vi "Send Query.vi"(8 "error in (no error)":errorcluster, 9 "Bytes Count":u32=1024, 10 "write buffer":string, 11 "VISA resource name":refnum<visa-resource-name>) -> (0 "error out":errorcluster, 2 "read buffer":string, 3 "VISA resource name out":refnum<visa-resource-name>)   [LabVIEW 2023, in "Anritsu Power Meter.lvlib"]
uses:
  Anritsu Power Meter.lvlib
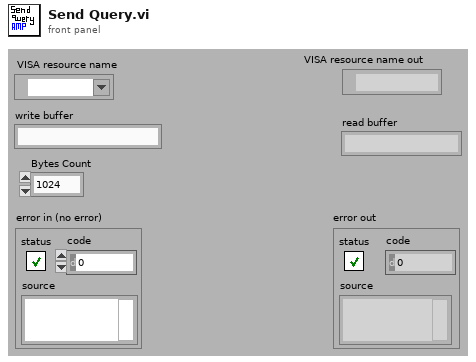
[diagram p1: front panel]
types:
  T1 = typedef "Semaphore RefNum" = refnum<k1>
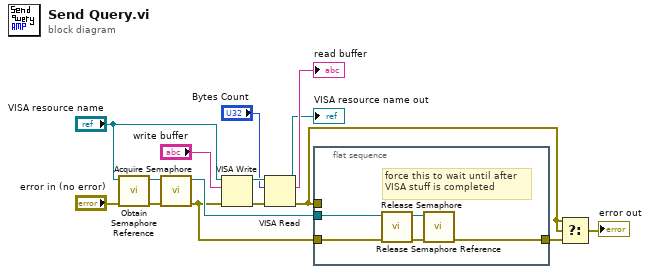
[diagram p0: block diagram]
diagram:
  n1 = call <vilib>:"Obtain Semaphore Reference.vi"("error in (no error)"="error in (no error)", "name (unnamed)"="VISA resource name") -> ("error out"=w10:errorcluster, "semaphore"=w11:T1)  [unwired: 1 in, 3 out]
  n2 = call <vilib>:"Acquire Semaphore.vi"("error in (no error)"=w10, "semaphore"=w11) -> ("error out"=w4:errorcluster, "semaphore out"=w8:T1)  [unwired: 1 in, 3 out]
  n3 = VISA Write(VISA resource name="VISA resource name", write buffer="write buffer", error in (no error)=w4) -> (VISA resource name out=w15:refnum<visa-resource-name>, error out=w13:errorcluster)  [unwired: 1 out]
  n4 = VISA Read(VISA resource name=w15, byte count="Bytes Count", error in (no error)=w13) -> (VISA resource name out=→"VISA resource name out":refnum<visa-resource-name>, read buffer=→"read buffer":string, error out=w3:errorcluster)  [unwired: 1 out]
  n5 = flat-sequence {
    tunnel: w8 -> [w20]
    tunnel: [w17] -> w5
    tunnel: w4 -> [w16]
    tunnel: w3 -> [_]
    frame #0 {
      # "force this to wait until after \nVISA stuff is completed"
      n6 = call <vilib>:"Release Semaphore.vi"("error in (no error)"=w16, "semaphore"=w20) -> ("error out"=w18:errorcluster, "semaphore out"=w19:T1)  [unwired: 4 out]
      n7 = call <vilib>:"Release Semaphore Reference.vi"("error in (no error)"=w18, "semaphore"=w19) -> ("error out"=w17:errorcluster)  [unwired: 9 out]
    }
  }
  n8 = Select(t=w3, s=w3, f=w5) -> (s? t:f=→"error out":errorcluster)
